vi "Error log.vi"(8 "error in (no error)":errorcluster) -> (0 "error in (no error) 2":errorcluster)   [LabVIEW 2018]
uses:
  Error log/Error log.lvclass
  C:/Users/Denis/Desktop/S4ACS/S4ACS/Log File/Log File.lvclass
  Log File/Log File.lvclass/Log File.ctl
  <vilib>/addons/_JKI Toolkits/Caraya/classes/Assert/Assert Not Error.vi
  <vilib>/addons/_JKI Toolkits/Caraya/classes/Assert/Assert Equal Value_Variant.vi
  <vilib>/addons/_JKI Toolkits/Caraya/classes/Test/Test.lvclass
  Log File/Log File.lvclass
  <vilib>/addons/_JKI Toolkits/Caraya/classes/Assert/Assert.lvclass
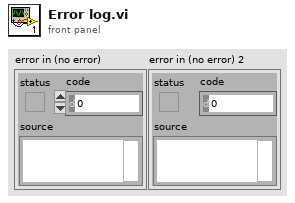
[diagram p1: front panel]
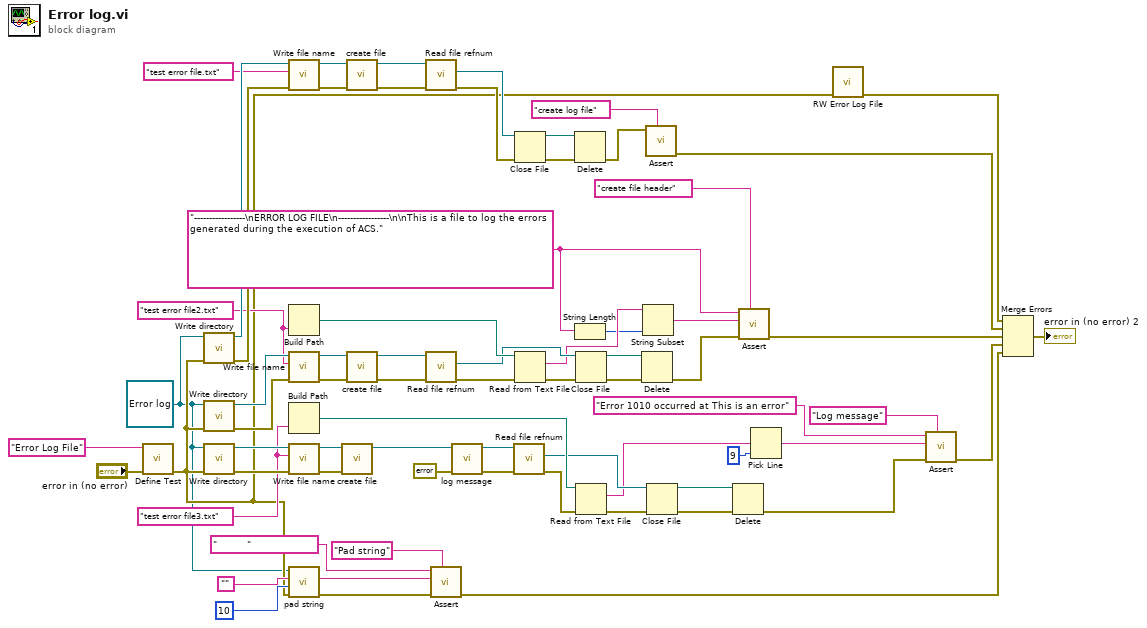
[diagram p0: block diagram]
diagram:
  w1 = "-----------------\nERROR LOG FILE\n-----------------\n\nThis is a file to log the errors generated during the execution of ACS." ("message of the file header")
  w7 = refnum<class "Error log.lvclass"> refnum ("Error log.lvclass")
  w29 = "test error file3.txt" ("file name")
  w44 = "test error file2.txt" ("file name")
  n1 = call <vilib>:"Define Test.vi"("error in (no error)"="error in (no error)", "Label (VI Title)"="Error Log File") -> ("error out"=w8:errorcluster)  [unwired: 8 in, 1 out]
  n2 = call "Write directory.vi"("error in (no error)"=w8, "Log File in"=w7) -> ("error out"=w65:errorcluster, "Log File out"=w64:refnum<class "Error log.lvclass">)  [unwired: 8 in]
  n3 = call "Write directory.vi"("error in (no error)"=w8, "Log File in"=w7) -> ("error out"=w51:errorcluster, "Log File out"=w50:refnum<class "Error log.lvclass">)  [unwired: 8 in]
  n4 = call "Write directory.vi"("error in (no error)"=w8, "Log File in"=w7) -> ("error out"=w34:errorcluster, "Log File out"=w33:refnum<class "Error log.lvclass">)  [unwired: 8 in]
  n5 = call "Write file name.vi"("error in (no error)"=w65, "suffix"="test error file.txt" ("file name"), "Log File in"=w64) -> ("error out"=w52:errorcluster, "Log File out"=w53:refnum<class "Error log.lvclass">)  [unwired: 7 in]
  n6 = Build Path(name or relative path=w44) -> (appended path=w43:path)  [unwired: 1 in]
  n7 = call "Write file name.vi"("error in (no error)"=w51, "suffix"=w44, "Log File in"=w50) -> ("error out"=w48:errorcluster, "Log File out"=w49:refnum<class "Error log.lvclass">)  [unwired: 7 in]
  n8 = Build Path(name or relative path=w29) -> (appended path=w30:path)  [unwired: 1 in]
  n9 = call "Write file name.vi"("error in (no error)"=w34, "suffix"=w29, "Log File in"=w33) -> ("error out"=w35:errorcluster, "Log File out"=w32:refnum<class "Error log.lvclass">)  [unwired: 7 in]
  n10 = call "pad string.vi"("error in (no error)"=w8, "string size"=u16 10, "input string"="", "Log File in"=w7) -> ("error out"=w9:errorcluster, "output string"=w13:string)  [unwired: 5 in, 1 out]
  n11 = call "create file.vi"("error in (no error)"=w35, "Log File in"=w32) -> ("Log File out"=w31:refnum<class "Error log.lvclass">)  [unwired: 8 in, 1 out]
  n12 = call "create file.vi"("error in (no error)"=w52, "Log File in"=w53) -> ("error out"=w55:errorcluster, "Log File out"=w54:refnum<class "Error log.lvclass">)  [unwired: 8 in]
  n13 = call "create file.vi"("error in (no error)"=w48, "Log File in"=w49) -> ("error out"=w47:errorcluster, "Log File out"=w46:refnum<class "Error log.lvclass">)  [unwired: 8 in]
  n14 = call "Read file refnum.vi"("error in (no error)"=w55, "Log File in"=w54) -> ("error out"=w59:errorcluster, "file refnum"=w56:refnum<file>)  [unwired: 7 in, 1 out]
  n15 = call "Read file refnum.vi"("error in (no error)"=w47, "Log File in"=w46) -> ("error out"=w45:errorcluster, "file refnum"=w36:refnum<file>)  [unwired: 7 in, 1 out]
  n16 = call-poly <vilib>:"Assert.vi"("Label"="Pad string" ("Label (VI Title)"), "error in (no error)"=w9, "Actual"=w13, "Expected"="          ") -> ("error out"=w10:errorcluster)  [unwired: 6 in, 1 out]
  n17 = call-dynamic "log message.vi"("error in (no error)"=errorcluster {"status"=TRUE, "code"=1010, "source"="This is an error"} ("error in (no error) 3"), "Error log in"=w31) -> ("error out"=w22:errorcluster, "Error log out"=w21:refnum<class "Error log.lvclass">)  [unwired: 8 in]
  n18 = call "Read file refnum.vi"("error in (no error)"=w22, "Log File in"=w21) -> ("error out"=w20:errorcluster, "file refnum"=w19:refnum<file>)  [unwired: 7 in, 1 out]
  n19 = Close File(refnum=w56, error in=w59) -> (path=w57:path, error out=w58:errorcluster)
  n20 = Read from Text File(file (use dialog)=w43, error in=w45) -> (text=w3:string, error out=w40:errorcluster)  [unwired: 2 in, 2 out]
  n21 = Delete(path (use dialog)=w57, error in=w58) -> (error out=w63:errorcluster)  [unwired: 3 in, 2 out]
  n22 = String Length(string=w1) -> (length=w2:i32)
  n23 = Close File(refnum=w36, error in=w40) -> (path=w38:path, error out=w41:errorcluster)
  n24 = Read from Text File(file (use dialog)=w30, error in=w20) -> (text=w17:string, error out=w26:errorcluster)  [unwired: 2 in, 2 out]
  n25 = Delete(path (use dialog)=w38, error in=w41) -> (error out=w39:errorcluster)  [unwired: 3 in, 2 out]
  n26 = String Subset(string=w3, length (rest)=w2) -> (substring=w4:string)  [unwired: 1 in]
  n27 = call-poly <vilib>:"Assert.vi"("Label"="create log file" ("Label (VI Title)"), "Not Error?"=w63) -> ("error out"=w62:errorcluster)  [unwired: 8 in, 1 out]
  n28 = Close File(refnum=w19, error in=w26) -> (path=w28:path, error out=w27:errorcluster)
  n29 = Delete(path (use dialog)=w28, error in=w27) -> (error out=w24:errorcluster)  [unwired: 3 in, 2 out]
  n30 = call-poly <vilib>:"Assert.vi"("Label"="create file header" ("Label (VI Title)"), "error in (no error)"=w39, "Actual"=w4, "Expected"=w1) -> ("error out"=w42:errorcluster)  [unwired: 6 in, 1 out]
  n31 = Pick Line(multi-line string=w17, line index=9) -> (output string=w5:string)  [unwired: 1 in]
  n32 = call "RW Error Log File.vi"("error in (no error)"=w8) -> ("error in (no error) 2"=w66:errorcluster)  [unwired: 10 in]
  n33 = call-poly <vilib>:"Assert.vi"("Label"="Log message" ("Label (VI Title)"), "error in (no error)"=w24, "Actual"=w5, "Expected"="Error 1010 occurred at This is an error" ("Label (VI Title)")) -> ("error out"=w25:errorcluster)  [unwired: 6 in, 1 out]
  n34 = Merge Errors(w66, w62, w42, w25, w10) -> (→"error in (no error) 2":errorcluster)
